vi "_FPGA_DDS_Quadrant.vi"(3 "RfCyc_in":u32) -> (0 "Cross?":bool, 1 "Quadrant":fxp<+,2,2>)   [LabVIEW 2018]
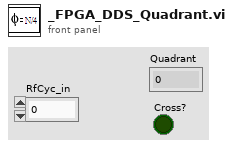
[diagram p1: front panel]
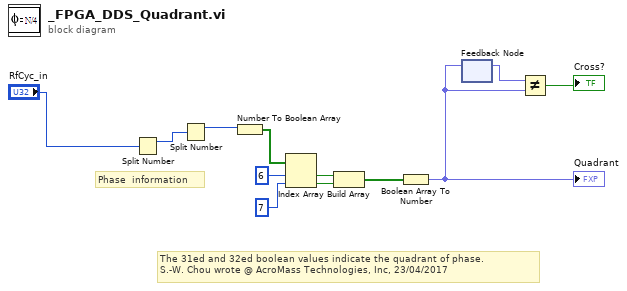
[diagram p0: block diagram]
diagram:
  # "The 31ed and 32ed boolean values indicate the quadrant of phase.\nS.-W. Chou wrote @ AcroMass Technologies, Inc, 23/04/2017"
  # "Phase  information"
  n1 = Split Number(x="RfCyc_in") -> (hi(x)=w12:u16)  [unwired: 1 out]
  n2 = Split Number(x=w12) -> (hi(x)=w5:u8)  [unwired: 1 out]
  n3 = Number To Boolean Array(number=w5) -> (Boolean array=w11:bool[])
  n4 = Index Array(array=w11, index #1=6 ("index"), index #2=7 ("index")) -> (element #1=w7:bool, element #2=w8:bool)
  n5 = Build Array(w7, w8) -> (w6:bool[])
  n6 = Boolean Array To Number(Boolean array=w6) -> (number=w3:fxp<+,2,2>)
  "Quadrant" <- w3
  n7 = feedback-in #1(w3) -> ()
  n8 = feedback #1() -> (w4:fxp<+,2,2>)  [unwired: 1 in]
  n9 = Not Equal?(x=w4, y=w3) -> (x != y?=→"Cross?":bool)
